vi "Global_OnCommand.vi"(10 "Command ID":string, 11 "Object":T1) -> ()   [LabVIEW 2020]
uses:
  <resource>/Framework/Providers/API/ItemRef.ctl
panel:
  out "error out":errorcluster
  in  "error in":errorcluster
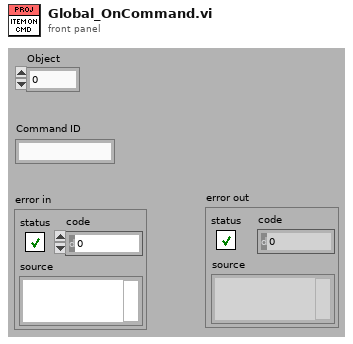
[diagram p1: front panel]
types:
  T1 = typedef "ItemRef.ctl" = u64
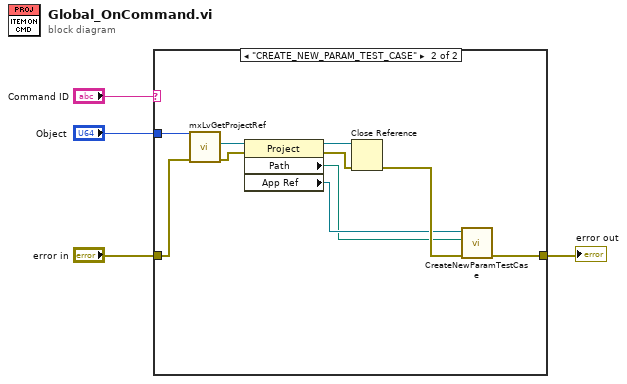
[diagram p0: block diagram]
diagram:
  n1 = case shown="\"CREATE_NEW_PARAM_TEST_CASE\"" "Command ID" {
    tunnel: "error in" -> [w5 w9]
    tunnel: [w5 w15] -> w2
    tunnel: "Object" -> [_ w10]
    frame Default {
    }
    frame "CREATE_NEW_PARAM_TEST_CASE" {
      n2 = call <resource>:"mxLvGetProjectRef.vi"("error in"=w9, "Item"=w10) -> ("error out"=w11:errorcluster, "Project Refnum"=w12:refnum<vi>)  [unwired: 7 in, 1 out]
      n3 = property class="Project"(reference=w12, error in=w11) -> (reference out=w13:refnum<vi>, error out=w14:errorcluster, "Path"=w6:path, "App Ref"=w7:refnum<vi>)
      n4 = Close Reference(reference=w13, error in (no error)=w14) -> (error out=w8:errorcluster)
      n5 = call "CreateNewParamTestCase.vi"("error in (no error)"=w8, "Path"=w6, "Application"=w7) -> ("error out"=w15:errorcluster)  [unwired: 8 in]
    }
  }
  "error out" <- w2
